vi "Get Enum Strings From File.vi"(8 "error in (no error)":errorcluster, 11 "EnumPath":path) -> (0 "error out":errorcluster, 3 "Strings []":string[](array[string]))   [LabVIEW 2020]
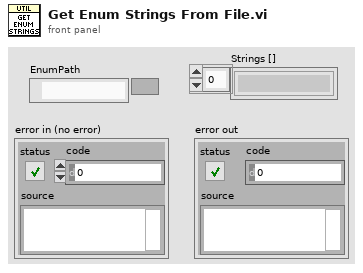
[diagram p1: front panel]
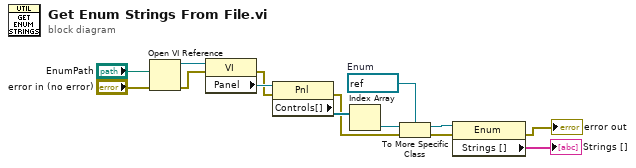
[diagram p0: block diagram]
diagram:
  w13 = refnum<vi> refnum  # Enum
  n1 = Open VI Reference(vi path="EnumPath", error in (no error)="error in (no error)") -> (vi reference=w9:refnum<vi>, error out=w5:errorcluster)  [unwired: 4 in]
  n2 = property class="VI"(reference=w9, error in=w5) -> (error out=w4:errorcluster, "Panel"=w11:refnum<vi>)  [unwired: 1 out]
  n3 = property class="Pnl"(reference=w11, error in=w4) -> (error out=w3:errorcluster, "Controls[]"=w10:refnum<vi>[])  [unwired: 1 out]
  n4 = Index Array(array=w10) -> (element=w12:refnum<vi>)  [unwired: 1 in]
  n5 = To More Specific Class(target class=w13, reference=w12, error in=w3) -> (specific class reference=w14:refnum<vi>, error out=w2:errorcluster)
  n6 = property class="Enum"(reference=w14, error in=w2) -> (error out=→"error out":errorcluster, "Strings []"=→"Strings []":string[])  [unwired: 1 out]
